vi "LogFileCloseRef.vi"(8 "error in (no error)":errorcluster, 10 "file":bool, 11 "Byte Stream File in":refnum<file>) -> (0 "error out":errorcluster, 3 "Byte Stream File out":refnum<file>)   [LabVIEW 2011]
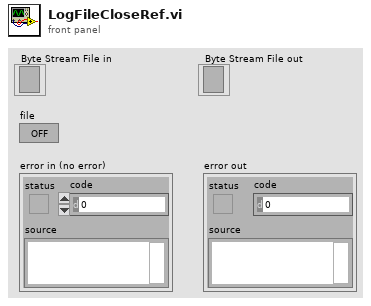
[diagram p1: front panel]
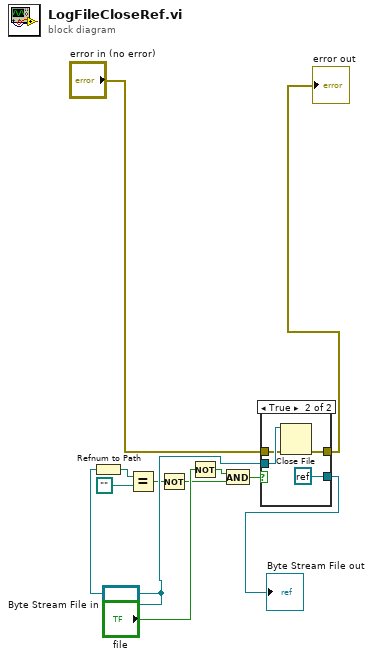
[diagram p0: block diagram]
diagram:
  n1 = Refnum to Path(1:"Byte Stream File in") -> (0:w5:path)
  n2 = Equal?(x=w5, y=path "") -> (x = y?=w3:bool)
  n3 = Not(x=w3) -> (.not. x?=w1:bool)
  n4 = Not(x="file") -> (.not. x?=w2:bool)
  n5 = And(x=w2, y=w1) -> (x .and. y?=w6:bool)
  n6 = case shown="True" w6 {
    tunnel: [w13 refnum<k0> refnum] -> w11
    tunnel: "Byte Stream File in" -> [w13 w17]
    tunnel: [w12 w16] -> w10
    tunnel: "error in (no error)" -> [w12 w14]
    frame False {
    }
    frame True {
      n7 = Close File(refnum=w17, error in=w14) -> (error out=w16:errorcluster)  [unwired: 1 out]
    }
  }
  "Byte Stream File out" <- w11
  "error out" <- w10
